vi "draw.f#g#a#.vi"(11 "midi-ui in":refnum<class "midi-ui.lvclass">) -> (2 "coordinates":cluster{"x":dbl, "y":dbl}[](array[cluster]), 3 "midi-ui out":refnum<class "midi-ui.lvclass">)   [LabVIEW 2020, in "midi-ui.lvclass"]
uses:
  midi-ui.lvclass
  midi-ui.lvclass/midi-ui.ctl
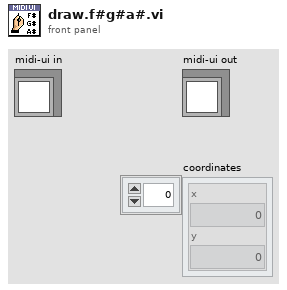
[diagram p1: front panel]
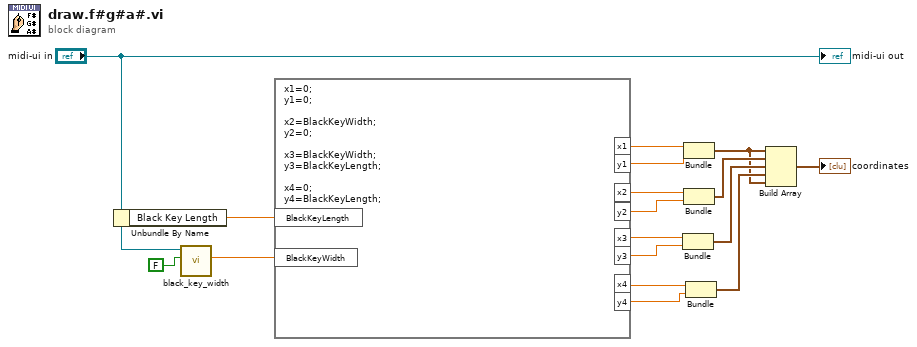
[diagram p0: block diagram]
diagram:
  n1 = Unbundle By Name("midi-ui in") -> ("Black Key Length"=w5:dbl)
  n2 = call "black_key_width.vi"("C# or D#?"=FALSE, "midi-ui in"="midi-ui in") -> ("Black Key Width"=w3:dbl)  [unwired: 8 in, 1 out]
  n3 = formula code="x1=0;\ny1=0;\n\nx2=BlackKeyWidth;\ny2=0;\n\nx3=BlackKeyWidth;\ny3=BlackKeyLength;\n\nx4=0;\ny4=BlackKeyLength;"("BlackKeyLength"=w5, "BlackKeyWidth"=w3) -> ("x1"=w17:dbl, "y1"=w16:dbl, "x2"=w10:dbl, "y2"=w11:dbl, "x3"=w12:dbl, "y3"=w15:dbl, "x4"=w13:dbl, "y4"=w14:dbl)
  n4 = Bundle("x3"=w12, "y3"=w15) -> (w8:cluster{"x3":dbl, "y3":dbl})  [unwired: 1 in]
  n5 = Bundle("x1"=w17, "y1"=w16) -> (w1:cluster{"x1":dbl, "y1":dbl})  [unwired: 1 in]
  n6 = Bundle("x2"=w10, "y2"=w11) -> (w9:cluster{"x2":dbl, "y2":dbl})  [unwired: 1 in]
  n7 = Bundle("x4"=w13, "y4"=w14) -> (w7:cluster{"x4":dbl, "y4":dbl})  [unwired: 1 in]
  n8 = Build Array(w1, w9, w8, w7, w1) -> (→"coordinates":cluster{"x1":dbl, "y1":dbl}[])
  "midi-ui out" <- "midi-ui in"
